vi "Resource from String.vi"(8 "error in (no error)":errorcluster, 10 "Resource from String":string, 11 "LC Parser in":refnum<class "LC Parser.lvclass">) -> (0 "error out":errorcluster, 2 "Resource as Variant":variant, 3 "LC Parser out":refnum<class "LC Parser.lvclass">)   [LabVIEW 2020, in "LC Parser.lvclass"]
uses:
  LC Parser.lvclass
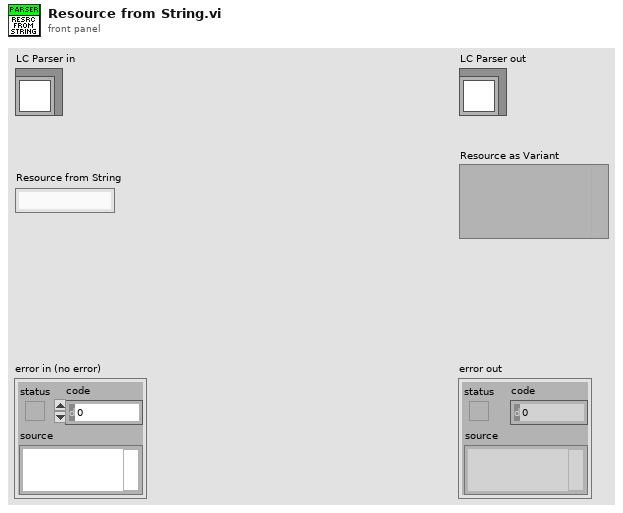
[diagram p1: front panel]
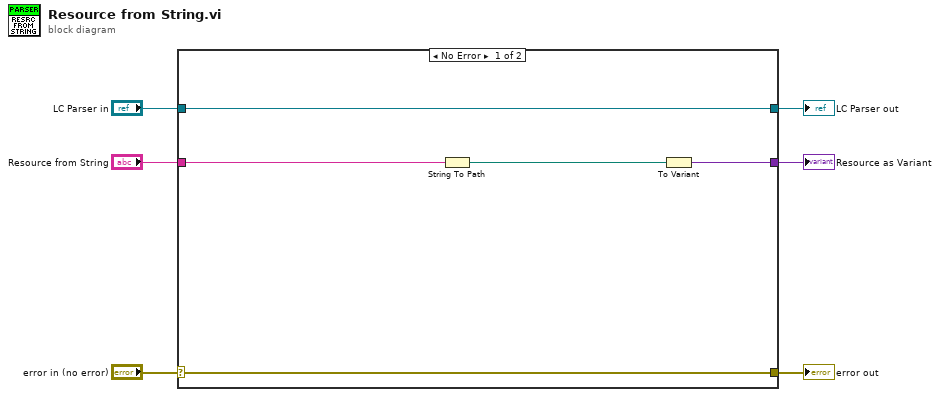
[diagram p0: block diagram]
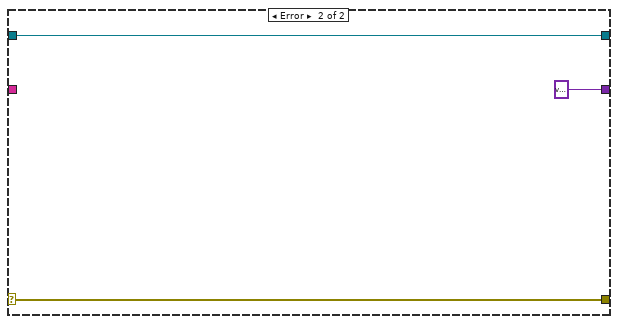
[diagram p2: hidden frame]
diagram:
  n1 = case shown="No Error" "error in (no error)" {
    selector: "error in (no error)" -> [w10 w14]
    tunnel: [w10 w14] -> w6
    tunnel: [w11 w13] -> w4
    tunnel: "LC Parser in" -> [w11 w13]
    tunnel: "Resource from String" -> [w9 _]
    tunnel: [w8 variant ("Resource as Variant")] -> w5
    frame No Error {
      n2 = String To Path(string=w9) -> (path=w7:path)
      n3 = To Variant(anything=w7) -> (Variant=w8:variant)
    }
    frame Error {
    }
  }
  "error out" <- w6
  "LC Parser out" <- w4
  "Resource as Variant" <- w5
